vi "QMH_Enqueue.vi"(4 "Priority? (F)":bool, 6 "Queue_Ref":T1, 7 "Flush (F)":bool, 8 "error in (no error)":errorcluster, 10 "Payload":variant, 11 "Message":string) -> (0 "error out":errorcluster)   [LabVIEW 2021, in "Framework_lib.lvlib"]
doc: "Enqueue element into the selected Queue"
uses:
  Framework_lib.lvlib
  QMH_references_enum.ctl
  framework_Qmessage.ctl
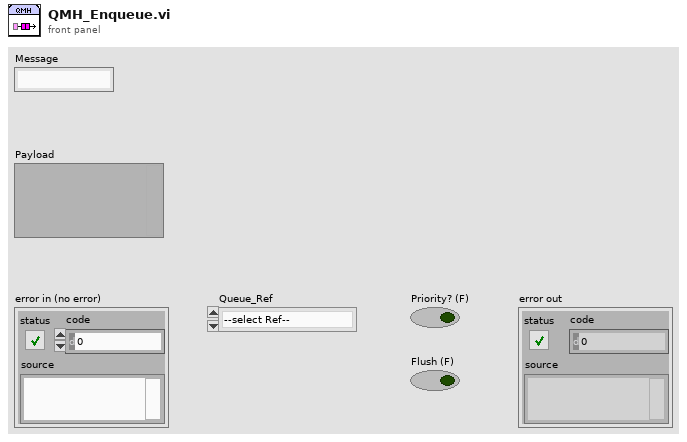
[diagram p1: front panel]
types:
  T1 = typedef "Framework_lib.lvlib/QMH_references_enum.ctl" = enum16{"--select Ref--", "Consumer_SUT", "Consumer_Annot", "Compute_Results"}
  T2 = typedef "Framework_lib.lvlib/framework_Qmessage.ctl" = cluster{"Message":string, "Payload":variant}
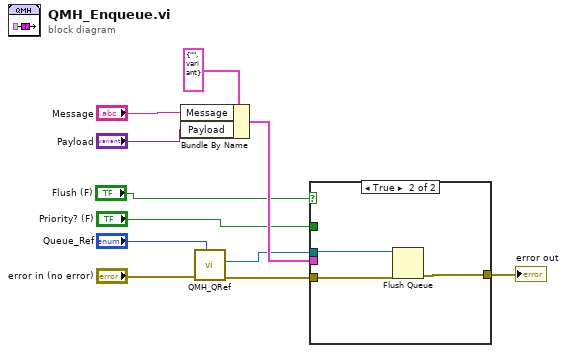
[diagram p0: block diagram]
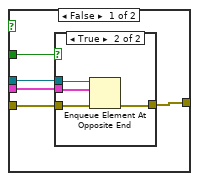
[diagram p2: hidden frame]
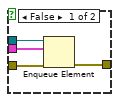
[diagram p3: hidden frame]
diagram:
  n1 = Bundle By Name(cluster=T2 {"Message"="", "Payload"=variant} ("element"), "Message"="Message", "Payload"="Payload") -> (w9:T2)
  n2 = call "QMH_QRef.vi"("Enum"="Queue_Ref", "error in (no error)"="error in (no error)") -> ("error out"=w7:errorcluster, "Queue_ref"=w4:refnum<queue>)  [unwired: 7 in, 1 out]
  n3 = case shown="True" "Flush (F)" {
    tunnel: [w16 w26] -> w11
    tunnel: w9 -> [w15 _]
    tunnel: w7 -> [w14 w27]
    tunnel: w4 -> [w13 w25]
    tunnel: "Priority? (F)" -> [w12 _]
    frame False {
      n4 = case shown="True" w12 {
        tunnel: [w20 w23] -> w16
        tunnel: w15 -> [w19 w22]
        tunnel: w14 -> [w18 w24]
        tunnel: w13 -> [w17 w21]
        frame False {
          n5 = Enqueue Element(queue=w17, element=w19, error in (no error)=w18) -> (error out=w20:errorcluster)  [unwired: 1 in, 2 out]
        }
        frame True {
          n6 = Enqueue Element At Opposite End(queue=w21, element=w22, error in (no error)=w24) -> (error out=w23:errorcluster)  [unwired: 1 in, 2 out]
        }
      }
    }
    frame True {
      n7 = Flush Queue(queue=w25, error in (no error)=w27) -> (error out=w26:errorcluster)  [unwired: 2 out]
    }
  }
  "error out" <- w11
